vi "Put Tracing Element In Array.vi"(2 "Y":dbl, 3 "X":dbl, 4 "InputTraceArray":dbl[][](array[numeric])) -> (0 "OutputTraceArray":dbl[][](array[numeric]), 1 "OutputXYElement":cluster{"X":dbl[], "Y":dbl[]})   [LabVIEW 2014]
panel:
  # "[x, y]"
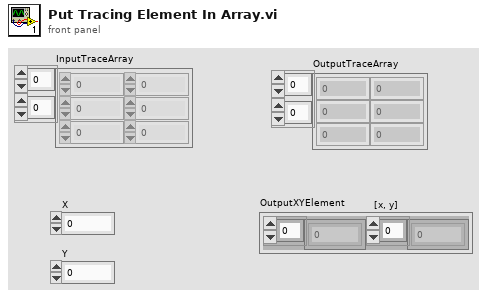
[diagram p1: front panel]
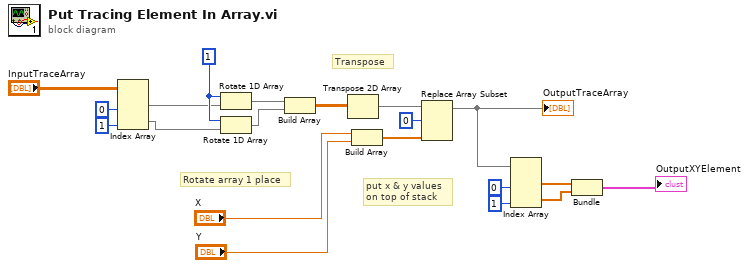
[diagram p0: block diagram]
diagram:
  w17 = 1 ("n")
  # "put x & y values\non top of stack"
  # "Transpose"
  # "Rotate array 1 place"
  n1 = Index Array(array="InputTraceArray", index (col) #1=0 ("disabled index (col)"), index (col) #2=1 ("index (col)")) -> (element #1=w16:dbl[], element #2=w15:dbl[])  [unwired: 2 in]
  n2 = Rotate 1D Array(1:w16, 2:w17) -> (0:w14:dbl[])
  n3 = Rotate 1D Array(1:w15, 2:w17) -> (0:w13:dbl[])
  n4 = Build Array(w14, w13) -> (w12:dbl[][])
  n5 = Transpose 2D Array(2D array=w12) -> (transposed array=w11:dbl[][])
  n6 = Build Array("X", "Y") -> (w3:dbl[])
  n7 = Replace Array Subset(array=w11, new element=w3, index (row)=0) -> (w7:dbl[][])  [unwired: 1 in]
  "OutputTraceArray" <- w7
  n8 = Index Array(array=w7, index (col) #1=0 ("disabled index (col)"), index (col) #2=1 ("index (col)")) -> (element #1=w6:dbl[], element #2=w5:dbl[])  [unwired: 2 in]
  n9 = Bundle(w6, w5) -> (→"OutputXYElement":cluster{dbl[], dbl[]})  [unwired: 1 in]
